vi "onGenerateNewInboundChannel.vi"(8 "error in (no error)":errorcluster, 11 "Connection.LocalQueue in":refnum<class "Connection.LocalQueue.lvclass">) -> (0 "error out":errorcluster, 3 "Connection.LocalQueue out":refnum<class "Connection.LocalQueue.lvclass">)   [LabVIEW 2013, in "Connection.Queue_GOSPL.lvlib" / "Connection.LocalQueue.lvclass"]
uses:
  Connection.LocalQueue.lvclass
  Connection/Connection.lvclass
  Connection/Connection.lvclass/Connection.ctl
  Connection.LocalQueue.lvclass/Connection.LocalQueue.ctl
  <vilib>/LabVIEW Open Source Project/Unicity/RandomStringGenerator/RandomStringGenerator.lvclass
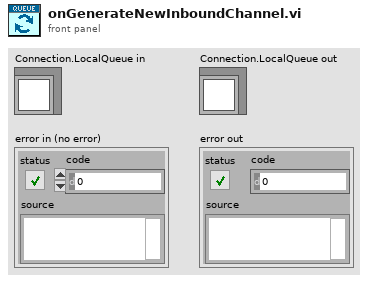
[diagram p1: front panel]
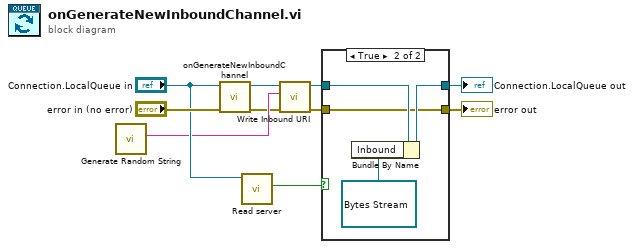
[diagram p0: block diagram]
diagram:
  n1 = call <vilib>:"Generate Random String.vi"() -> ("Random String"=w6:string)  [unwired: 11 in]
  n2 = call-parent "onGenerateNewInboundChannel.vi"("error in (no error)"="error in (no error)", "Connection in"="Connection.LocalQueue in") -> ("error out"=w3:errorcluster, "Connection out"=w8:refnum<class "Connection.LocalQueue.lvclass">)  [unwired: 8 in]
  n3 = call "Read server.vi"("Connection in"="Connection.LocalQueue in") -> ("server"=w4:bool)  [unwired: 9 in, 1 out]
  n4 = call "Write Inbound URI.vi"("Inbound URI"=w6, "Connection in"=w8) -> ("Connection out"=w5:refnum<class "Connection.LocalQueue.lvclass">)  [unwired: 9 in]
  n5 = case shown="True" w4 {
    tunnel: w5 -> [w11 w15]
    tunnel: w3 -> [w10 w13]
    tunnel: [w11 w14] -> w2
    tunnel: [w10 w13] -> w1
    frame False {
    }
    frame True {
      n6 = Bundle By Name(cluster=w15, "Inbound"=refnum<queue> refnum) -> (w14:refnum<class "Connection.LocalQueue.lvclass">)
    }
  }
  "error out" <- w1
  "Connection.LocalQueue out" <- w2
